vi "Lucky_Number.vi"(0 "Application_Directory":path, 11 "Error_In":errorcluster) -> (15 "Error_Out":errorcluster)   [LabVIEW 2021]
doc: "This is a VI work as one of the front panel of the Game, Showing the user their Lucky Number."
uses:
  Controls/State.ctl
  <vilib>/numeric/Random Number (Range) U64.vi
  Controls/Bool_Button.ctl
panel:
  out "Lucky_Number_Out":string
  in  "Home":T1
  in  "Back?":T1
  in  "Next?":T1
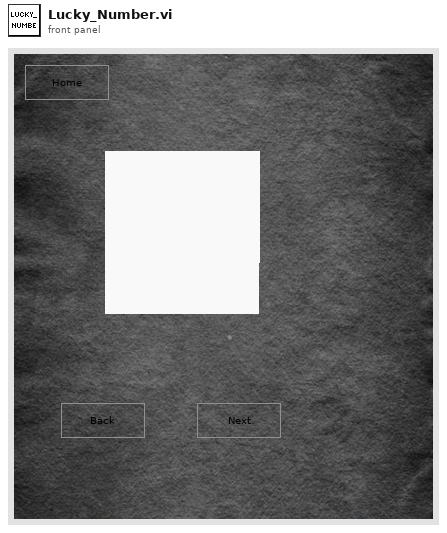
[diagram p1: front panel]
types:
  T1 = typedef "Bool_Button.ctl" = bool
  T2 = enum32{"Invalid", "Standard", "Closed", "Hidden", "Minimized", "Maximized"}
  T3 = typedef "State.ctl" = enum16{"Close", "Password_Popup", "Start_Popup", "Wizard_Msg", "Get_Name_DoB", "Lucky_Number", "Q-1", "Q-2", "Q-3", "Nature_of_the_Person"}
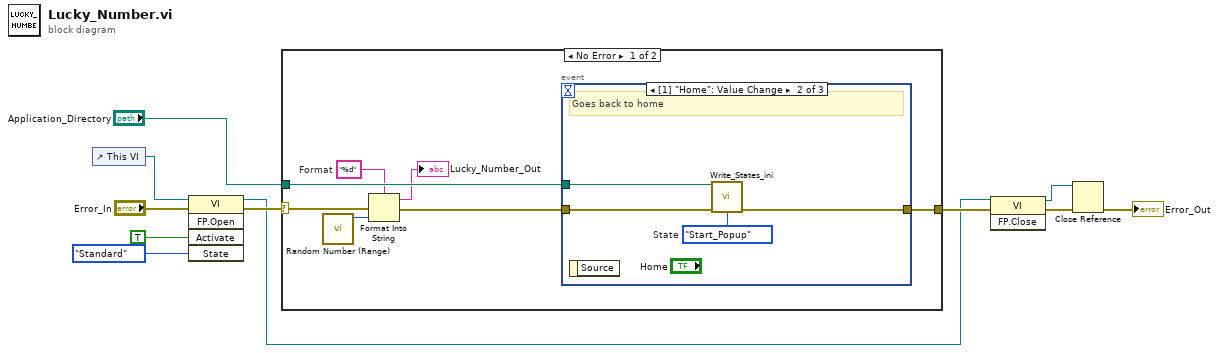
[diagram p0: block diagram]
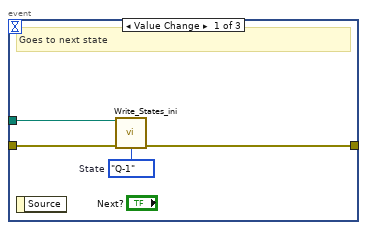
[diagram p2: hidden frame]
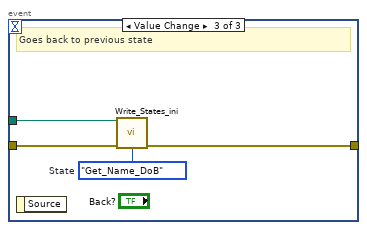
[diagram p3: hidden frame]
diagram:
  n1 = control-ref of="This VI"() -> (w9:refnum<vi>)
  n2 = invoke class="VI" method="FP.Open"(reference=w9, error in="Error_In", "Activate"=TRUE ("Activate?"), "State"=T2."Standard") -> (reference out=w1:refnum<vi>, error out=w10:errorcluster)  [unwired: 1 in, 3 out]
  n3 = case shown="No Error" w10 {
    selector: w10 -> [w12 w31]
    tunnel: [w18 w31] -> w3
    tunnel: "Application_Directory" -> [w17 _]
    frame No Error {
      w14 = "%d"  # Format
      n4 = call-poly <vilib>:"Random Number (Range).vi"() -> ("number"=w16:u64)  [unwired: 11 in]
      n5 = Format Into String(format string=w14, error in=w12, w16) -> (resulting string=→"Lucky_Number_Out":string, error out=w13:errorcluster)  [unwired: 1 in]
      n6 = event shown="[1] \"Home\": Value Change" {
        selector: _ -> [_ _ _]
        dyn-events: _ -> [_ _ _]
        timeout: _ -> [_ _ _]
        tunnel: w13 -> [w21 w26 w30]
        tunnel: [w22 w25 w29] -> w18
        tunnel: w17 -> [w19 w23 w27]
        event Value Change {
          w20 = State."Q-1"  # State
          # "Goes to next state"
          n7 = event-data() -> ()  [unwired: 1 in, 1 out]
          n8 = call "Write_States_ini.vi"("Application_Directory"=w19, "Error_In"=w21, "State"=w20) -> ("Error_Out"=w22:errorcluster)  [unwired: 12 in]
        }
        event Value Change {
          w24 = State."Start_Popup"  # State
          # "Goes back to home"
          n9 = event-data() -> ()  [unwired: 1 in, 1 out]
          n10 = call "Write_States_ini.vi"("Application_Directory"=w23, "Error_In"=w26, "State"=w24) -> ("Error_Out"=w25:errorcluster)  [unwired: 12 in]
        }
        event Value Change {
          w28 = State."Get_Name_DoB"  # State
          # "Goes back to previous state"
          n11 = event-data() -> ()  [unwired: 1 in, 1 out]
          n12 = call "Write_States_ini.vi"("Application_Directory"=w27, "Error_In"=w30, "State"=w28) -> ("Error_Out"=w29:errorcluster)  [unwired: 12 in]
        }
      }
    }
    frame Error {
    }
  }
  n13 = invoke class="VI" method="FP.Close"(reference=w1, error in=w3) -> (reference out=w6:refnum<vi>, error out=w5:errorcluster)  [unwired: 1 in, 1 out]
  n14 = Close Reference(reference=w6, error in (no error)=w5) -> (error out=→"Error_Out":errorcluster)
